vi "Check Cal Stimulus Params.vi"(8 "error in (no error)":errorcluster, 11 "Cal Stimulus":T1={"Min Freq (Hz)"=50.0, "Max Freq (Hz)"=50000.0, "Freq Step (Hz)"=50.0, "Waveform"=enum."Chirp", "Attenuation (dB)"=20.0, "Sample Rate (Hz)"=100000.0}) -> (0 "error out":errorcluster)   [LabVIEW 2020]
uses:
  Type Defs/Cal Stimulus.ctl
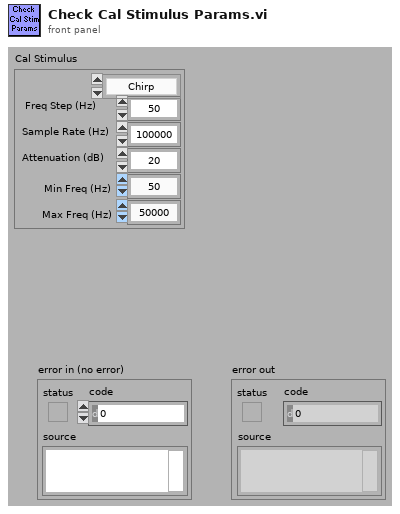
[diagram p1: front panel]
types:
  T1 = typedef "Cal Stimulus.ctl" = cluster{"Min Freq (Hz)":dbl, "Max Freq (Hz)":dbl, "Freq Step (Hz)":dbl, "Waveform":enum16{"Chirp", "Weighted"}, "Attenuation (dB)":dbl, "Sample Rate (Hz)":dbl}
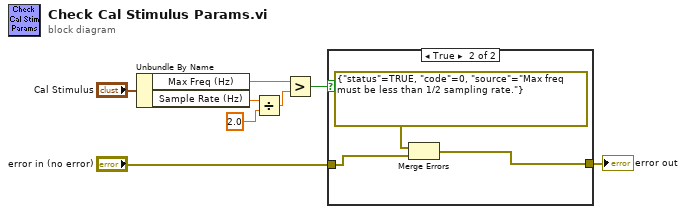
[diagram p0: block diagram]
diagram:
  n1 = Unbundle By Name("Cal Stimulus") -> ("Max Freq (Hz)"=w7:dbl, "Sample Rate (Hz)"=w6:dbl)
  n2 = Divide(x=w6, y=2.0) -> (x/y=w4:dbl)
  n3 = Greater?(x=w7, y=w4) -> (0:w3:bool)
  n4 = case shown="True" w3 {
    tunnel: "error in (no error)" -> [w9 w11]
    tunnel: [w9 w12] -> w1
    frame False {
    }
    frame True {
      n5 = Merge Errors(errorcluster {"status"=TRUE, "code"=0, "source"="Max freq must be less than 1/2 sampling rate."} ("error in 1 (no error)"), w11) -> (w12:errorcluster)
    }
  }
  "error out" <- w1
